vi "CThread Get Iteration Index.vi"   [LabVIEW 2012, in "CThread.lvlib"]
uses:
  CThread.lvlib
  XNodes/terminalnode/CThread VI Terminal Node.xnode
  Base/CThread Base - Get Iteration Index.vi
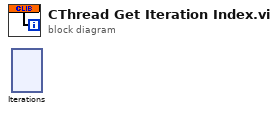
[diagram p0: block diagram]
diagram:
  n1 = xnode "Iterations"() -> ()  [unwired: 1 in, 2 out]
